vi "ex6.vi"() -> ()   [LabVIEW 2022 SP3]
panel:
  in  "Numeric 10":dbl
  in  "Numeric 9":dbl
  in  "Numeric 8":dbl
  in  "Numeric 7":dbl
  in  "Numeric 6":dbl
  in  "Numeric 5":dbl
  in  "Numeric 4":dbl
  in  "Numeric 3":dbl
  in  "Numeric 2":dbl
  in  "Numeric":dbl
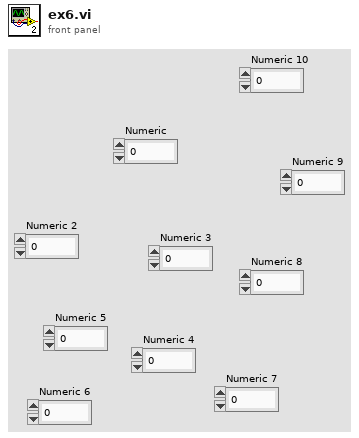
[diagram p1: front panel]
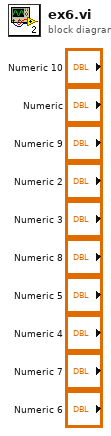
[diagram p0: block diagram]
diagram:
